vi "batchgenkey.vi"(0 "MoAgSy_GPG in":refnum<class "MoAgSy_GPG.lvclass">, 1 "options file":path, 2 "keyringfile":path, 3 "Sec keyringfile":path, 4 "password":string, 5 "error in (no error)":errorcluster, 6 "Name":string, 8 "Trust DB":path) -> (10 "dup Trust DB":path, 12 "Key-ID":string, 13 "success":bool, 14 "MoAgSy_GPG out":refnum<class "MoAgSy_GPG.lvclass">, 15 "dup options file":path, 16 "dup keyringfile":path, 17 "dup Sec keyringfile":path, 19 "error out":errorcluster)   [LabVIEW 2009, in "MoAgSy.lvlib" / "MoAgSy_GPG.lvclass"]
doc: "Generate a Key with a batch command. If no Password is set, the function uses a self-created. If no Name is set, the object's name will is used."
uses:
  MoAgSy_GPG.lvclass
  HGF_GPG/HGF_GPG.lvclass/HGF_GPG.lvclass
panel:
  out "Error?":bool[](array[boolean])
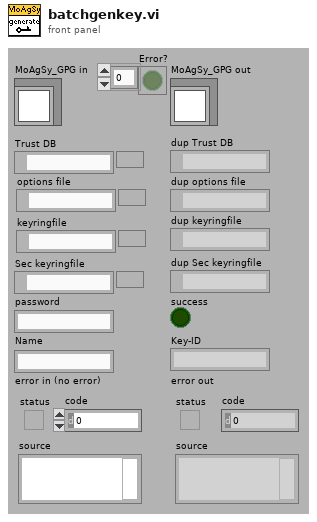
[diagram p1: front panel]
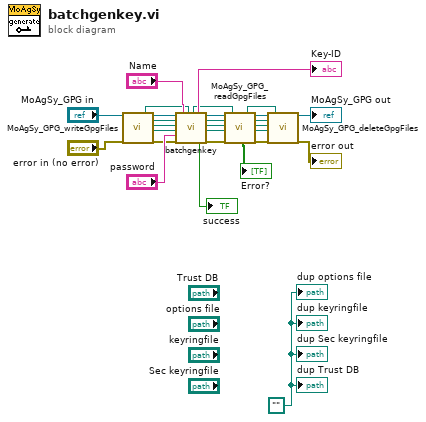
[diagram p0: block diagram]
diagram:
  w4 = path ""
  n1 = call "MoAgSy_GPG_writeGpgFiles.vi"("MoAgSy_GPG"="MoAgSy_GPG in", "error in (no error)"="error in (no error)") -> ("trust db file"=w12:path, "dup MoAgSy_GPG"=w16:refnum<class "MoAgSy_GPG.lvclass">, "options file"=w15:path, "keyring file"=w14:path, "sec keyring file"=w13:path, "error out"=w1:errorcluster)  [unwired: 12 out]
  n2 = call-parent "batchgenkey.vi"("HGF_GPG in"=w16, "options file"=w15, "keyringfile"=w14, "Sec keyringfile"=w13, "password"="password", "error in (no error)"=w1, "Name"="Name", "Trust DB"=w12) -> ("dup Trust DB"=w5:path, "Key-ID"=→"Key-ID":string, "success"=→"success":bool, "HGF_GPG out"=w6:refnum<class "MoAgSy_GPG.lvclass">, "dup options file"=w9:path, "dup keyringfile"=w8:path, "dup Sec keyringfile"=w7:path, "error out"=w3:errorcluster)  [unwired: 4 out]
  n3 = call "MoAgSy_GPG_readGpgFiles.vi"("MoAgSy_GPG in"=w6, "options file"=w9, "keyring file"=w8, "sec keyring file"=w7, "error in (no error)"=w3, "trust db file"=w5) -> ("Error?"=→"Error?":bool[], "dup trust db file"=w18:path, "MoAgSy_GPG out"=w24:refnum<class "MoAgSy_GPG.lvclass">, "dup options file"=w23:path, "dup keyring file"=w22:path, "dup sec keyring file"=w21:path, "error out"=w20:errorcluster)  [unwired: 7 out]
  n4 = call "MoAgSy_GPG_deleteGpgFiles.vi"("MoAgSy_GPG"=w24, "options file"=w23, "keyringfile"=w22, "Sec keyringfile"=w21, "error in (no error)"=w20, "Trust DB"=w18) -> ("dup MoAgSy_GPG"=→"MoAgSy_GPG out":refnum<class "MoAgSy_GPG.lvclass">, "error out"=→"error out":errorcluster)  [unwired: 12 out]
  "dup options file" <- w4
  "dup keyringfile" <- w4
  "dup Sec keyringfile" <- w4
  "dup Trust DB" <- w4
